vi "Stop Core.vi"(10 "final error code":i32, 11 "Nested in":refnum<class "Thermometer Multichannel Worker.lvclass">) -> (3 "Nested out":refnum<class "Thermometer Multichannel Worker.lvclass">)   [LabVIEW 2024, in "Thermometer Multichannel Worker.lvlib" / "Thermometer Multichannel Worker.lvclass"]
doc: "(<B>Filename</B>: Actor Framework.lvlib:Actor.lvclass:Stop Core.vi)\n\nDefines what the actor does before it stops. Use the <B>final error code</B> input to determine whether the actor shut down in response to an error.\n\nBy default, this method does nothing. A descendant class may override it to define behavior, such as shutting down any processes the actor initiated in its override of the Actor Core method."
uses:
  Thermometer Multichannel Worker.lvclass
  Thermometer Multichannel Worker.lvclass/Thermometer Multichannel Worker.ctl
  <vilib>/ActorFramework/Actor/Actor.lvclass
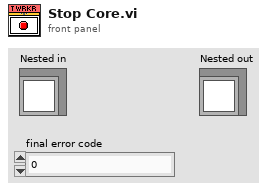
[diagram p1: front panel]
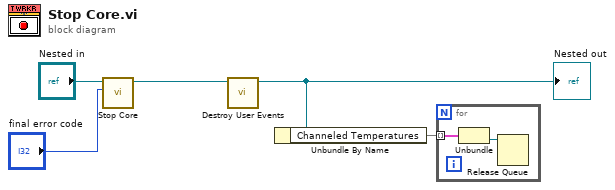
[diagram p0: block diagram]
diagram:
  n1 = call-parent "Stop Core.vi"("final error code"="final error code", "Actor in"="Nested in") -> ("Actor out"=w3:refnum<class "Thermometer Multichannel Worker.lvclass">)  [unwired: 9 in]
  n2 = call "Destroy User Events.vi"("UI Template in"=w3) -> ("UI Template out"=w2:refnum<class "Thermometer Multichannel Worker.lvclass">)  [unwired: 10 in]
  "Nested out" <- w2
  n3 = Unbundle By Name(w2) -> ("Channeled Temperatures"=w1:map{string, refnum<queue>})
  n4 = for {
    tunnel: w1 -> [w7] mode=indexing
    n5 = Unbundle(w7) -> ("WAV Queue"=w6:refnum<queue>)  [unwired: 1 out]
    n6 = Release Queue(queue=w6) -> ()  [unwired: 2 in, 3 out]
  }
